vi "_AnalyzeErrors.vi"() -> ()   [LabVIEW 2012]
uses:
  <userlib>/ROSforLV/ROS/Code/SubVIs/_ROSControl.ctl
  <userlib>/ROSforLV/ROS/Code/SubVIs/_ROSDirection.ctl
panel:
  in  "Delete Errors?":bool
  out "Cluster":T1
  in  "stop":bool
  in  "Tab Control":T2(tab)
  out "Console Errors":T5(array[cluster])
  out "ServerErrors":T5(array[cluster])
  out "servers qn":T5(array[cluster])
  out "servers v2d":T5(array[cluster])
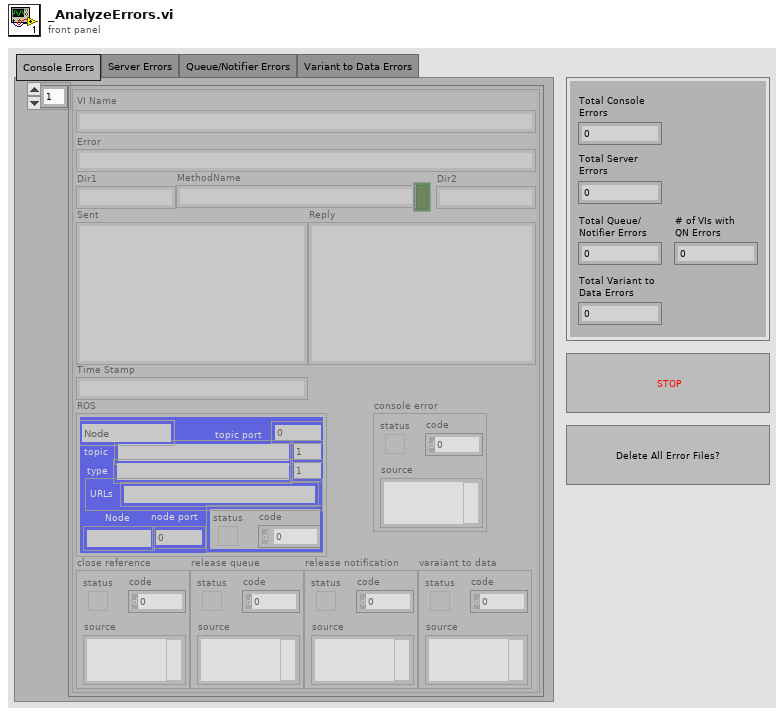
[diagram p1: front panel]
types:
  T1 = cluster{"Total Server\nErrors":i32, "Total Variant to\nData Errors":i32, "Total Queue/\nNotifier Errors":i32, "# of VIs with\nQN Errors":i32, "Total Console\nErrors":i32}
  T2 = enum32{"Console Errors", "Server Errors", "Queue/Notifier Errors", "Variant to Data Errors"}
  T3 = typedef "_ROSControl.ctl" = cluster{"topic port":u16, "Node":string, "topic":string, "type":string, "node port":u32, "error ":errorcluster, "Direction":T4, "APIs":string[], "Update (ms)":u16, "write queue":u16}
  T4 = typedef "_ROSDirection.ctl" = enum16{"Node", "Publisher", "Subscriber", "Service Client"}
  T5 = cluster{"Sent":string, "Reply":string, "MethodName":string, "success":bool, "Dir1":string, "Dir2":string, "Error":string, "VI Name":string, "ROS":T3, "close reference":errorcluster, "release queue":errorcluster, "release notification":errorcluster, "varaiant to data":errorcluster, "console error":errorcluster, "Time Stamp":string}[]
  T6 = cluster{"Console":cluster{"Sent":string, "Reply":string, "MethodName":string, "success":bool, "Dir1":string, "Dir2":string, "Error":string, "VI Name":string, "ROS":T3, "close reference":errorcluster, "release queue":errorcluster, "release notification":errorcluster, "varaiant to data":errorcluster, "console error":errorcluster, "Time Stamp":string}[], "Server":cluster{"Sent":string, "Reply":string, "MethodName":string, "success":bool, "Dir1":string, "Dir2":string, "Error":string, "VI Name":string, "ROS":T3, "close reference":errorcluster, "release queue":errorcluster, "release notification":errorcluster, "varaiant to data":errorcluster, "console error":errorcluster, "Time Stamp":string}[], "QN":cluster{"Sent":string, "Reply":string, "MethodName":string, "success":bool, "Dir1":string, "Dir2":string, "Error":string, "VI Name":string, "ROS":T3, "close reference":errorcluster, "release queue":errorcluster, "release notification":errorcluster, "varaiant to data":errorcluster, "console error":errorcluster, "Time Stamp":string}[], "V2D":cluster{"Sent":string, "Reply":string, "MethodName":string, "success":bool, "Dir1":string, "Dir2":string, "Error":string, "VI Name":string, "ROS":T3, "close reference":errorcluster, "release queue":errorcluster, "release notification":errorcluster, "varaiant to data":errorcluster, "console error":errorcluster, "Time Stamp":string}[]}
  T7 = cluster{"Sent":string, "Reply":string, "Method Name":string, "success":bool, "Dir1":string, "Dir2":string, "Error Information":string, "VI Name":string, "ROS":T3, "close reference":errorcluster, "release queue":errorcluster, "release notification":errorcluster, "varaiant to data":errorcluster, "console error":errorcluster, "Time Stamp":string}
  T8 = cluster{"Sent":string, "Reply":string, "Method Name":string, "success":bool, "Dir1":string, "Dir2":string, "Error Information":string, "VI Name":string, "ROS":T3, "close reference":errorcluster, "release queue":errorcluster, "release notification":errorcluster, "varaiant to data":errorcluster, "console error":errorcluster, "Time Stamp":string}[]
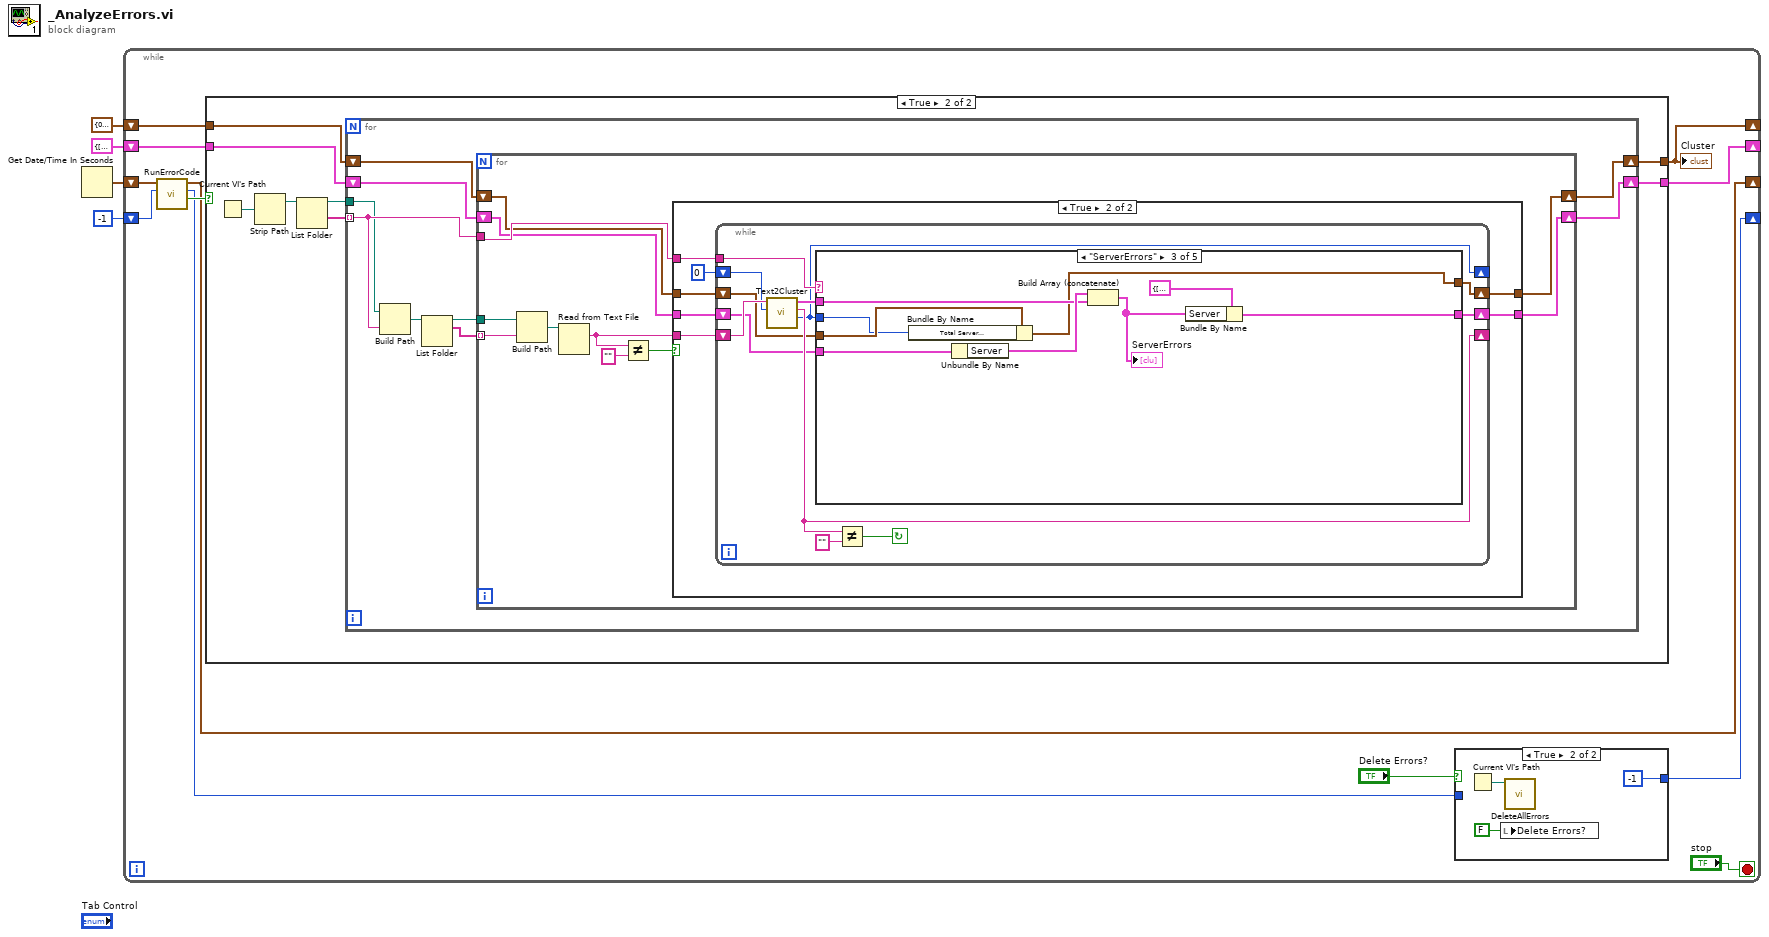
[diagram p0: block diagram]
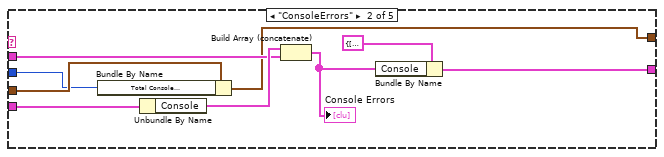
[diagram p6: hidden frame]
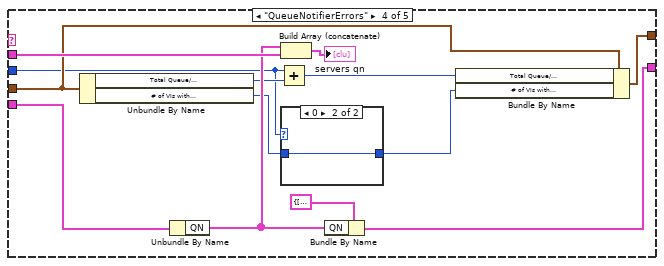
[diagram p7: hidden frame]
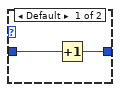
[diagram p8: hidden frame]
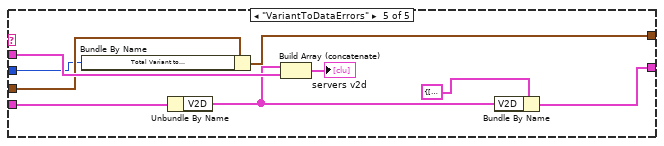
[diagram p9: hidden frame]
diagram:
  n1 = Get Date/Time In Seconds() -> (seconds since 1Jan1904=w2:timestamp)
  n2 = while {
    shift-right: [w14] -> _
    shift-left: T6 {"Console"=[], "Server"=[], "QN"=[], "V2D"=[]} -> [w15]
    shift-right: [w12] -> _
    shift-left: T1 {"Total Server\nErrors"=0, "Total Variant to\nData Errors"=0, "Total Queue/\nNotifier Errors"=0, "# of VIs with\nQN Errors"=0, "Total Console\nErrors"=0} ("Cluster") -> [w13]
    shift-right: [w8] -> _
    shift-left: w2 -> [w10]
    shift-right: [w5] -> _
    shift-left: -1 -> [w11]
    stop <- "stop" stop-if-true
    n3 = call <userlib>:"RunErrorCode.vi"("previous #"=w11, "previous time"=w10) -> ("Run"=w9:bool, "Number of Error Files"=w6:i32, "current time"=w8:timestamp)  [unwired: 7 in]
    n4 = case shown="True" w9 {
      tunnel: w15 -> [w21 w26]
      tunnel: [w21 w25] -> w14
      tunnel: w13 -> [w22 w24]
      tunnel: [w22 w23] -> w12
      frame False {
      }
      frame True {
        n5 = Current VI's Path() -> (path=w29:path)
        n6 = Strip Path(path=w29) -> (stripped path=w28:path)  [unwired: 1 out]
        n7 = List Folder(path=w28) -> (path out=w27:path, folder names=w30:string[])  [unwired: 3 in, 2 out]
        n8 = for {
          tunnel: w30 -> [w39] mode=indexing
          tunnel: w27 -> [w38]
          shift-right: [w33] -> w25
          shift-left: w26 -> [w34]
          shift-right: [w31] -> w23
          shift-left: w24 -> [w32]
          n9 = Build Path(base path=w38, name or relative path=w39) -> (appended path=w37:path)
          n10 = List Folder(path=w37) -> (path out=w35:path, filenames=w36:string[])  [unwired: 3 in, 2 out]
          n11 = for {
            tunnel: w39 -> [w50]
            tunnel: w36 -> [w49] mode=indexing
            tunnel: w35 -> [w48]
            shift-right: [w45] -> w33
            shift-left: w34 -> [w46]
            shift-right: [w43] -> w31
            shift-left: w32 -> [w44]
            n12 = Build Path(base path=w48, name or relative path=w49) -> (appended path=w47:path)
            n13 = Read from Text File(file (use dialog)=w47) -> (text=w41:string)  [unwired: 3 in, 3 out]
            n14 = Not Equal?(x=w41, y="") -> (x != y?=w42:bool)
            n15 = case shown="True" w42 {
              tunnel: w50 -> [_ w59]
              tunnel: w41 -> [_ w58]
              tunnel: w46 -> [w51 w57]
              tunnel: [w51 w56] -> w45
              tunnel: w44 -> [w52 w55]
              tunnel: [w52 w54] -> w43
              frame False {
              }
              frame True {
                n16 = while {
                  tunnel: w59 -> [w71]
                  shift-right: [w68] -> _
                  shift-left: w58 -> [w70]
                  shift-right: [w64] -> w56
                  shift-left: w57 -> [w65]
                  shift-right: [w62] -> w54
                  shift-left: w55 -> [w63]
                  shift-right: [w60] -> _
                  shift-left: 0 ("# of Errors") -> [w61]
                  stop <- w69 continue-if-true
                  n17 = call <userlib>:"Text2Cluster.vi"("Errors In"=w61, "string"=w70) -> ("# of Errors"=w60:i32, "remainder"=w68:string, "Log"=w66:T7)  [unwired: 7 in]
                  n18 = case shown="\"ServerErrors\"" w71 {
                    tunnel: w66 -> [_ w80 w90 w103 w114]
                    tunnel: w65 -> [w73 w82 w89 w104 w115]
                    tunnel: [w73 w77 w86 w99 w111] -> w64
                    tunnel: w63 -> [w72 w76 w85 w97 w110]
                    tunnel: w60 -> [_ w74 w84 w92 w108]
                    tunnel: [w72 w75 w83 w98 w109] -> w62
                    frame Default {
                    }
                    frame "ConsoleErrors" {
                      n19 = Bundle By Name(cluster=w76, "Total Console\nErrors"=w74) -> (w75:T1)
                      n20 = Unbundle By Name(w82) -> ("Console"=w81:T5)
                      n21 = Build Array (concatenate)(w81, w80) -> (w78:T8)
                      "Console Errors" <- w78
                      n22 = Bundle By Name(cluster=T6 {"Console"=[], "Server"=[], "QN"=[], "V2D"=[]}, "Console"=w78) -> (w77:T6)
                    }
                    frame "ServerErrors" {
                      n23 = Bundle By Name(cluster=w85, "Total Server\nErrors"=w84) -> (w83:T1)
                      n24 = Unbundle By Name(w89) -> ("Server"=w91:T5)
                      n25 = Build Array (concatenate)(w91, w90) -> (w87:T8)
                      "ServerErrors" <- w87
                      n26 = Bundle By Name(cluster=T6 {"Console"=[], "Server"=[], "QN"=[], "V2D"=[]}, "Server"=w87) -> (w86:T6)
                    }
                    frame "QueueNotifierErrors" {
                      n27 = Unbundle By Name(w97) -> ("Total Queue/\nNotifier Errors"=w94:i32, "# of VIs with\nQN Errors"=w96:i32)
                      n28 = Unbundle By Name(w104) -> ("QN"=w100:T5)
                      n29 = Add(x=w92, y=w94) -> (x+y=w93:i32)
                      n30 = Build Array (concatenate)(w100, w103) -> (→"servers qn":T8)
                      n31 = case shown="0" w92 {
                        tunnel: w96 -> [w106 w107]
                        tunnel: [w105 w107] -> w95
                        frame Default {
                          n32 = Increment(x=w106) -> (x+1=w105:i32)
                        }
                        frame 0 {
                        }
                      }
                      n33 = Bundle By Name(cluster=T6 {"Console"=[], "Server"=[], "QN"=[], "V2D"=[]}, "QN"=w100) -> (w99:T6)
                      n34 = Bundle By Name(cluster=w97, "Total Queue/\nNotifier Errors"=w93, "# of VIs with\nQN Errors"=w95) -> (w98:T1)
                    }
                    frame "VariantToDataErrors" {
                      n35 = Bundle By Name(cluster=w110, "Total Variant to\nData Errors"=w108) -> (w109:T1)
                      n36 = Unbundle By Name(w115) -> ("V2D"=w112:T5)
                      n37 = Build Array (concatenate)(w112, w114) -> (→"servers v2d":T8)
                      n38 = Bundle By Name(cluster=T6 {"Console"=[], "Server"=[], "QN"=[], "V2D"=[]}, "V2D"=w112) -> (w111:T6)
                    }
                  }
                  n39 = Not Equal?(x=w68, y="") -> (x != y?=w69:bool)
                }
              }
            }
          }
        }
      }
    }
    "Cluster" <- w12
    n40 = case shown="True" "Delete Errors?" {
      tunnel: [w17 -1 ("Number of Error Files")] -> w5
      tunnel: w6 -> [w17 _]
      frame False {
      }
      frame True {
        n41 = Current VI's Path() -> (path=w18:path)
        n42 = local write "Delete Errors?"(FALSE ("Delete Errors?")) -> ()
        n43 = call <userlib>:"DeleteAllErrors.vi"("path"=w18) -> ()  [unwired: 11 in]
      }
    }
  }
